vi "Actor Core.vi"(8 "error in":cluster{"状态":bool, "代码":i32, "源":string} caption="错误输入", 11 "蒸发冷却器":refnum<class "Evaporative Cooler.lvclass">) -> (0 "error out":cluster{"状态":bool, "代码":i32, "源":string} caption="错误输出", 3 "操作者输出":refnum<class "Actor.lvclass">)   [LabVIEW 2015, in "Evaporative Cooler.lvlib" / "Evaporative Cooler.lvclass"]
doc: "Actor Core.vi包含操作者的主要消息处理循环。操作者通常位于该循环中，在各种消息到达时对消息进行处理。如Do.vi消息返回任何错误，该循环将停止运行，错误代码43将被作为“无错误停止”的标准信号发送给调用方。如需更改上述行为，可在子孙类的Handle Error.vi中对该部分逻辑进行重写。"
uses:
  Evaporative Cooler.lvclass
  <vilib>/ActorFramework/Actor/Actor.lvclass
  Cooler Update Fan Status Msg/Cooler Update Fan Status Msg.lvclass
  Cooler Update Water Level Msg/Cooler Update Water Level Msg.lvclass
  Timed Loop Actor/Timed Loop Actor/Timed Loop Actor.lvclass/Timed Loop Actor.ctl
  Dual Fan/Dual Fan/Dual Fan.lvclass/Dual Fan.ctl
  Water Level/Water Level.lvclass/Water Level.ctl
  Evaporative Cooler.lvclass/Evaporative Cooler.ctl
  <vilib>/Utility/LVClass/Get LV Class Path.vi
  Cooler/Cooler/Cooler.lvclass
  Dual Fan/Dual Fan/Dual Fan.lvclass
  Level Controller/Level Controller/Level Controller.lvclass
  Timed Loop Actor/Timed Loop Actor/Timed Loop Actor.lvclass
  Water Level/Water Level.lvclass
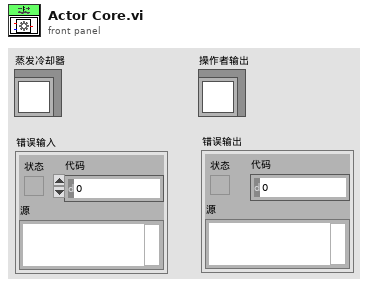
[diagram p1: front panel]
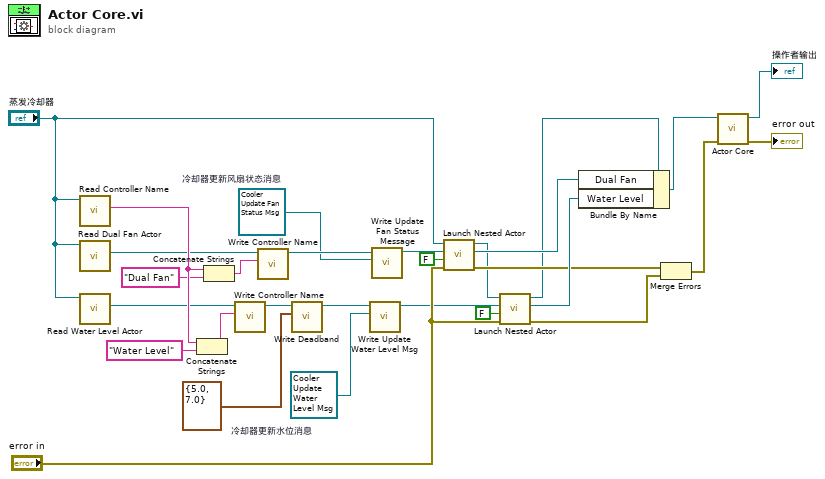
[diagram p0: block diagram]
diagram:
  w9 = refnum<class "Cooler Update Water Level Msg.lvclass"> refnum  # 冷却器更新水位消息
  w14 = refnum<class "Cooler Update Fan Status Msg.lvclass"> refnum  # 冷却器更新风扇状态消息
  n1 = call "Read Controller Name.vi"("定时循环控制器"="蒸发冷却器") -> ("控制器名称"=w18:string)  [unwired: 10 in]
  n2 = call-dynamic "Read Dual Fan Actor.vi"("蒸发冷却器"="蒸发冷却器") -> ("双风扇"=w13:refnum<class "Dual Fan.lvclass">)  [unwired: 10 in]
  n3 = call-dynamic "Read Water Level Actor.vi"("蒸发冷却器"="蒸发冷却器") -> ("水位"=w12:refnum<class "Water Level.lvclass">)  [unwired: 10 in]
  n4 = Concatenate Strings(w18, "Water Level" ("string")) -> (w19:string)
  n5 = Concatenate Strings(w18, "Dual Fan" ("string")) -> (w15:string)
  n6 = call "Write Controller Name.vi"("控制器名称"=w19, "定时循环控制器输入"=w12) -> ("定时循环控制器输出"=w11:refnum<class "Water Level.lvclass">)  [unwired: 9 in]
  n7 = call "Write Controller Name.vi"("控制器名称"=w15, "定时循环控制器输入"=w13) -> ("定时循环控制器输出"=w20:refnum<class "Dual Fan.lvclass">)  [unwired: 9 in]
  n8 = call "Write Deadband.vi"("死区"=cluster{"LO":dbl, "HI":dbl} {"LO"=5.0, "HI"=7.0} ("Deadband"), "水位控制器输入"=w11) -> ("水位控制器输出"=w10:refnum<class "Water Level.lvclass">)  [unwired: 8 in, 1 out]
  n9 = call "Write Update Water Level Msg.vi"("更新水位消息"=w9, "水位输入"=w10) -> ("水位输出"=w6:refnum<class "Water Level.lvclass">)  [unwired: 9 in]
  n10 = call "Write Update Fan Status Message.vi"("更新消息"=w14, "双风扇输入"=w20) -> ("双风扇输出"=w7:refnum<class "Dual Fan.lvclass">)  [unwired: 9 in]
  n11 = call <vilib>:"Launch Nested Actor.vi"("error in (no error)"="error in", "Auto-stop? (T)"=FALSE, "Nested Actor"=w7, "Caller Actor in"="蒸发冷却器") -> ("error out"=w24:errorcluster, "Nested Actor's Enqueuer"=w26:refnum<class "Message Enqueuer.lvclass">, "Caller Actor out"=w5:refnum<class "Evaporative Cooler.lvclass">)  [unwired: 5 in]
  n12 = call <vilib>:"Launch Nested Actor.vi"("error in (no error)"="error in", "Auto-stop? (T)"=FALSE, "Nested Actor"=w6, "Caller Actor in"=w5) -> ("error out"=w23:errorcluster, "Nested Actor's Enqueuer"=w27:refnum<class "Message Enqueuer.lvclass">, "Caller Actor out"=w3:refnum<class "Evaporative Cooler.lvclass">)  [unwired: 5 in]
  n13 = Bundle By Name(cluster=w3, "Dual Fan"=w26, "Water Level"=w27) -> (w25:refnum<class "Evaporative Cooler.lvclass">)
  n14 = Merge Errors(w24, w23) -> (w22:errorcluster)
  n15 = call-parent "Actor Core.vi"("error in"=w22, "定时循环控制器"=w25) -> ("error out"=→"error out":cluster{"状态":bool, "代码":i32, "源":string}, "操作者输出"=→"操作者输出":refnum<class "Actor.lvclass">)  [unwired: 8 in]
